vi "control_style.vi"() -> ()   [LabVIEW 2015, in "lv-blog-interface-prototype.lvlib"]
uses:
  lv-blog-interface-prototype.lvlib
panel:
  out "vertical_progress_bar":dbl(slide) scale=0.0..100.0
  out "horizontal_progress_bar":dbl(slide) scale=0.0..100.0
  in  "filepath":path
  in  "exit":bool
  in  "string":string
  in  "navigation":enum32{"No Selection", "tool", "build"}(radio)=enum."tool"
  out "tab_control":enum32{"Tool", "Build"}(tab)
  in  "tree":string[](tree)
  in  "boolean":bool
  # "Controls we'll use:\n* string indicator/control\n* button\n* tree\n* tab control\n* file path control (for configuration)\n* button dialog (for navigation)\n* progress bar"
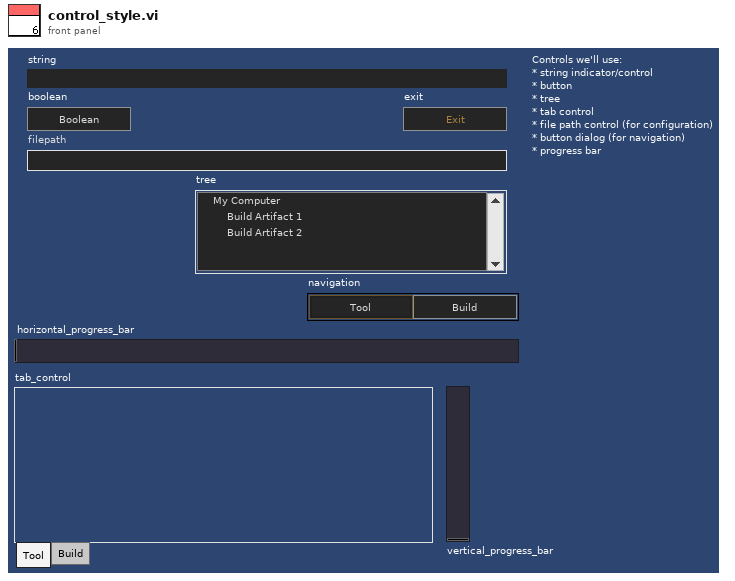
[diagram p1: front panel]
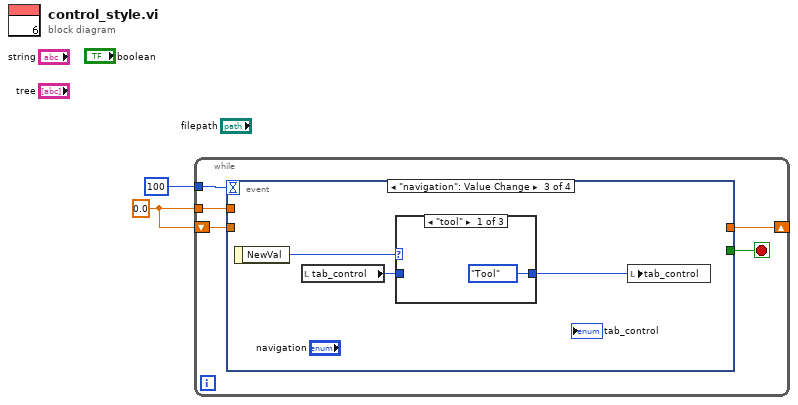
[diagram p0: block diagram]
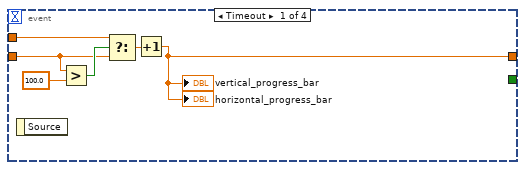
[diagram p2: hidden frame]
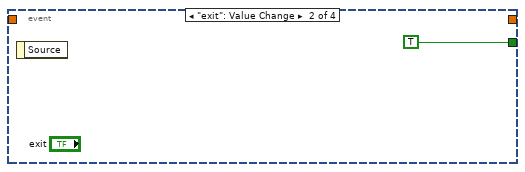
[diagram p3: hidden frame]
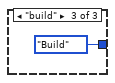
[diagram p5: hidden frame]
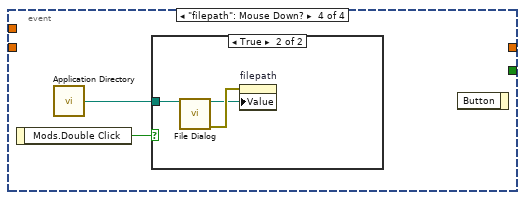
[diagram p6: hidden frame]
diagram:
  w1 = 0.0
  n1 = while {
    tunnel: 100 -> [w6]
    shift-right: [w4] -> _
    shift-left: w1 -> [w5]
    tunnel: w1 -> [w3]
    stop <- w7 stop-if-true
    n2 = event shown="[2] \"navigation\": Value Change" {
      selector: _ -> [_ _ _ _]
      dyn-events: _ -> [_ _ _ _]
      timeout: w6 -> [_ _ _ _]
      tunnel: [_ TRUE _ _] -> w7
      tunnel: w5 -> [w10 _ _ _]
      tunnel: [w8 _ _ _] -> w4
      tunnel: w3 -> [w11 _ _ _]
      event Timeout {
        n3 = event-data() -> ()  [unwired: 1 in, 1 out]
        n4 = Greater?(x=w10, y=100.0) -> (0:w12:bool)
        n5 = Select(t=w11, s=w12, f=w10) -> (s? t:f=w9:dbl)
        n6 = Increment(x=w9) -> (x+1=w8:dbl)
        "vertical_progress_bar" <- w8
        "horizontal_progress_bar" <- w8
      }
      event "exit": Value Change {
        n7 = event-data() -> ()  [unwired: 1 in, 1 out]
      }
      event "navigation": Value Change {
        n8 = event-data() -> ("NewVal"=w17:enum32{"No Selection", "tool", "build"})  [unwired: 1 in]
        n9 = local read "tab_control"() -> (w16:enum32{"Tool", "Build"})
        n10 = case shown="\"tool\"" w17 {
          tunnel: w16 -> [_ w19 _]
          tunnel: [enum32{"Tool", "Build"}."Tool" ("tab_control") w19 enum32{"Tool", "Build"}."Build" ("tab_control")] -> w15
          frame "tool" {
          }
          frame Default {
          }
          frame "build" {
          }
        }
        n11 = local write "tab_control"(w15) -> ()
      }
      event "filepath": Mouse Down? {
        n12 = event-data() -> ("Mods.Double Click"=w22:bool)  [unwired: 1 in]
        n13 = call <vilib>:"Application Directory.vi"() -> ("Application Directory"=w21:path)
        n14 = case shown="True" w22 {
          tunnel: w21 -> [_ w23]
          frame False {
          }
          frame True {
            n15 = call "File Dialog"("start path"=w23) -> ("selected path"=w24:path, "error out"=w25:errorcluster)  [unwired: 11 in, 2 out]
            n16 = property on="filepath" class="Path"(error in=w25, "Value"=w24) -> ()  [unwired: 1 in, 2 out]
          }
        }
        n17 = event-data() -> ()  [unwired: 2 in, 1 out]
      }
    }
  }
